vi "SLSC Write Properties.vi"(0 "session in":refnum<k21>, 1 "Stop Updating?":bool, 3 "Detect?":bool[](array[boolean]), 5 "SLSC Module Name":refnum<k21>, 9 "Values":dbl[](array[numeric]), 11 "error in":errorcluster, 12 "SLSC Dynamic Outputs":T1[](array[typedef])) -> (4 "session out":refnum<k21>, 6 "SLSC Module Name":refnum<k21>, 8 "LoopRate(ms)":u32=50, 15 "error out":errorcluster)   [LabVIEW 2015, in "SLSC CD Engine.lvlib"]
uses:
  SLSC CD Engine.lvlib
  SLSC Dynamic Channel.ctl
  SLSC Datatype.ctl
  <vilib>/SLSC/Commit Properties for Devices.vi
  <vilib>/SLSC/Set Generic Property (U64).vi
  <vilib>/SLSC/Set Generic Property (U32).vi
  <vilib>/SLSC/Set Generic Property (String).vi
  <vilib>/SLSC/Set Generic Property (I64).vi
  <vilib>/SLSC/Set Generic Property (I32).vi
  <vilib>/SLSC/Set Generic Property (DBL).vi
  <vilib>/SLSC/Set Generic Property (Bool).vi
  <vilib>/SLSC/SLSC.lvlib
  <vilib>/NI VeriStand/Custom Device Tools/Custom Device Utility Library/Custom Device Utility Library.lvlib
  SLSC CD Shared/SLSC CD Shared.lvlib
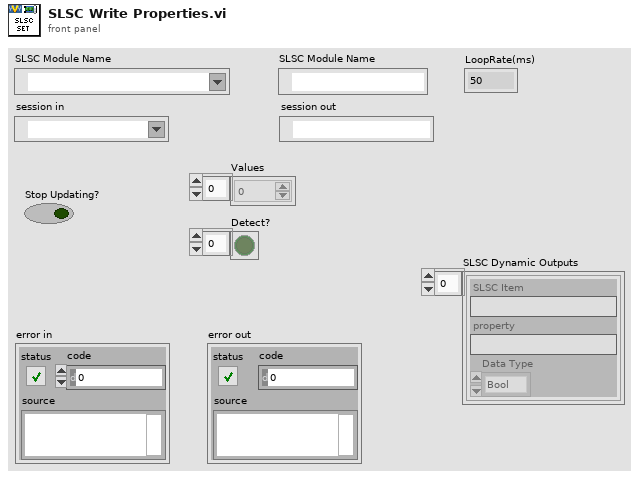
[diagram p1: front panel]
types:
  T1 = typedef "SLSC CD Shared.lvlib/SLSC Dynamic Channel.ctl" = cluster{"SLSC Item":string, "property":string, "Data Type":T2}
  T2 = typedef "SLSC CD Shared.lvlib/SLSC Datatype.ctl" = enum16{"Bool", "Double", "I32", "I64", "String", "U32", "U64"}
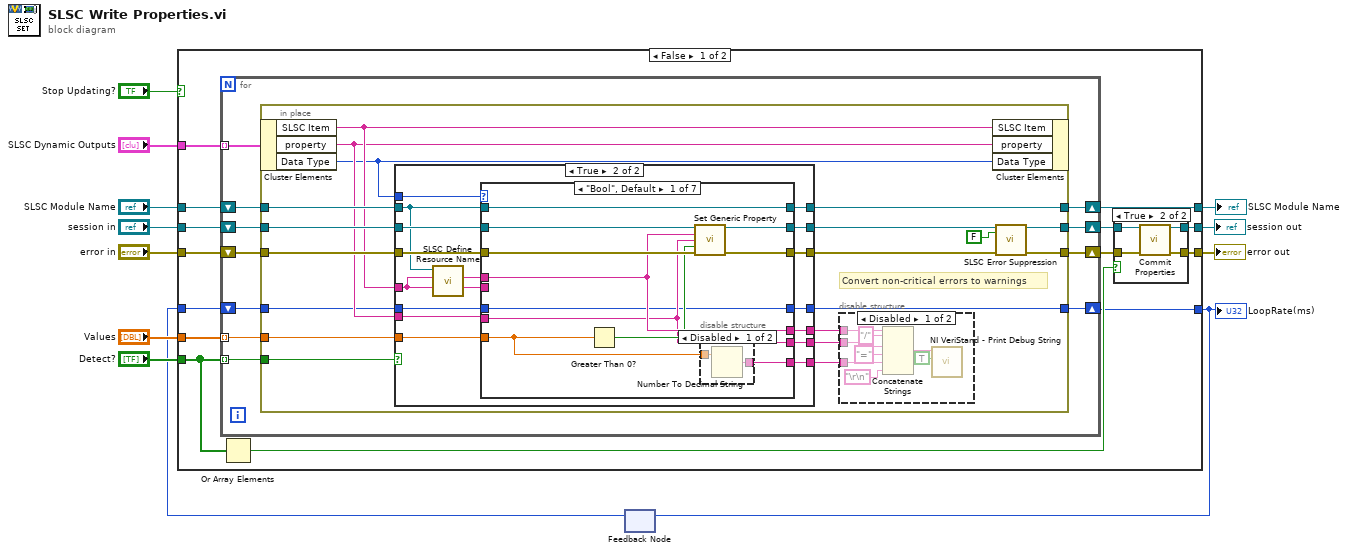
[diagram p0: block diagram]
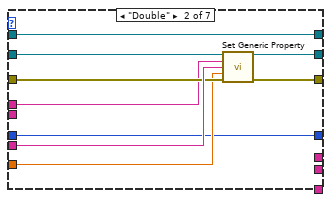
[diagram p6: hidden frame]
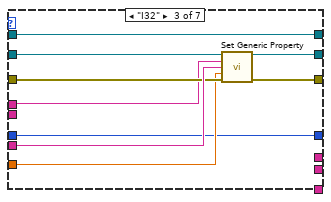
[diagram p7: hidden frame]
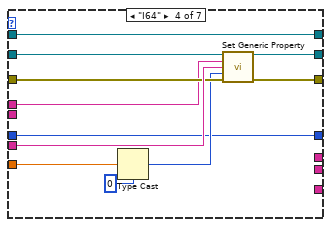
[diagram p8: hidden frame]
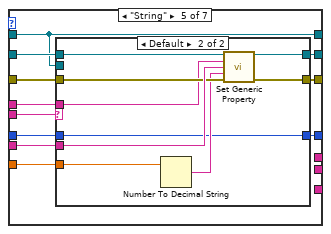
[diagram p9: hidden frame]
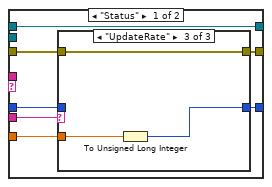
[diagram p10: hidden frame]
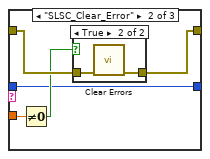
[diagram p12: hidden frame]
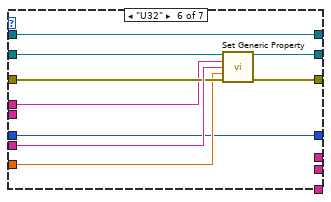
[diagram p14: hidden frame]
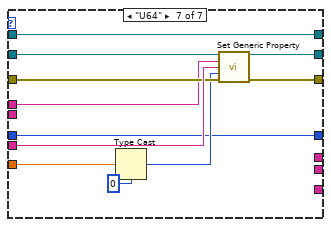
[diagram p15: hidden frame]
diagram:
  n1 = feedback #1() -> (w1:u32)  [unwired: 1 in]
  n2 = case shown="False" "Stop Updating?" {
    tunnel: "error in" -> [w26 w193]
    tunnel: "SLSC Dynamic Outputs" -> [w25 _]
    tunnel: "Values" -> [w24 _]
    tunnel: "session in" -> [w23 w194]
    tunnel: "SLSC Module Name" -> [w22 w195]
    tunnel: [w21 w195] -> w8
    tunnel: [w19 w193] -> w7
    tunnel: [w17 w194] -> w6
    tunnel: "Detect?" -> [w16 _]
    tunnel: [w13 w192] -> w2
    tunnel: w1 -> [w14 w192]
    frame False {
      n3 = for {
        tunnel: w24 -> [w43] mode=indexing
        tunnel: w25 -> [w36] mode=indexing
        shift-right: [w41] -> w18
        shift-left: w23 -> [w42]
        shift-right: [w40] -> w21
        shift-left: w22 -> [w37]
        tunnel: w16 -> [w35] mode=indexing
        shift-right: [w33] -> w13
        shift-left: w14 -> [w34]
        shift-right: [w38] -> w20
        shift-left: w26 -> [w39]
        n4 = in-place {
          in-place-border: w43 -> [w53]
          in-place-border: w42 -> [w61]
          in-place-border: [w60] -> w41
          in-place-border: [w59] -> w40
          in-place-border: w39 -> [w58]
          in-place-border: [w44] -> w38
          in-place-border: w37 -> [w57]
          in-place-border: w35 -> [w49]
          in-place-border: [w47] -> w33
          in-place-border: w34 -> [w46]
          # "Convert non-critical errors to warnings"
          n5 = in-place-cluster #2(w36) -> ("SLSC Item"=w56:string, "property"=w55:string, "Data Type"=w54:T2)
          n6 = case shown="True" w49 {
            tunnel: w61 -> [w72 w89]
            tunnel: [w72 w88] -> w60
            tunnel: [w73 w87] -> w59
            tunnel: w58 -> [w71 w86]
            tunnel: [w71 w85] -> w48
            tunnel: w57 -> [w73 w84]
            tunnel: w56 -> [_ w82]
            tunnel: w55 -> [_ w81]
            tunnel: w54 -> [_ w80]
            tunnel: w53 -> [_ w79]
            tunnel: [_ w78] -> w52
            tunnel: [_ w77] -> w51
            tunnel: [_ w76] -> w50
            tunnel: [w70 w75] -> w47
            tunnel: w46 -> [w70 w74]
            frame False {
            }
            frame True {
              n7 = call "SLSC Define Resource Name.vi"("SLSC Item"=w82, "SLSC Module Name"=w84) -> ("Resource"=w83:string)  [unwired: 9 in]
              n8 = case shown="\"Bool\", Default" w80 {
                tunnel: w79 -> [w95 w105 w114 w125 w137 w174 w184]
                tunnel: w89 -> [w100 w111 w120 w131 w142 w180 w191]
                tunnel: [w99 w110 w119 w130 w141 w179 w190] -> w88
                tunnel: w81 -> [w92 w109 w118 w129 w140 w178 w189]
                tunnel: w84 -> [w98 w108 w117 w128 w136 w177 w188]
                tunnel: [w98 w108 w117 w128 w136 w177 w188] -> w87
                tunnel: w86 -> [w97 w107 w116 w127 w139 w176 w187]
                tunnel: [w96 w106 w115 w126 w138 w175 w186] -> w85
                tunnel: w83 -> [w94 w104 w113 w122 w134 w173 w182]
                tunnel: w82 -> [_ _ _ _ w135 _ _]
                tunnel: [w94 _ _ _ _ _ _] -> w78
                tunnel: [w92 _ _ _ _ _ _] -> w77
                tunnel: [w91 _ _ _ _ _ _] -> w76
                tunnel: [w90 w103 w112 w121 w133 w172 w181] -> w75
                tunnel: w74 -> [w90 w103 w112 w121 w132 w172 w181]
                frame "Bool", Default {
                  n9 = Greater Than 0?(x=w95) -> (x > 0?=w93:bool)
                  n10 = call-poly <vilib>:"Set Generic Property.vi"("session in"=w100, "resources"=w94, "property"=w92, "property value"=w93, "error in (no error)"=w97) -> ("session out"=w99:refnum<k21>, "error out"=w96:errorcluster)  [unwired: 9 in]
                  n11 = disable-structure shown="Disabled" {
                    disable-tunnel: w95 -> [w102 _]
                    disable-tunnel: [w101 _] -> w91
                    frame Disabled {
                      n12 = Number To Decimal String(number=w102) -> (decimal integer string=w101:string)  [unwired: 1 in]
                    }
                    frame Enabled {
                    }
                  }
                }
                frame "Double" {
                  n13 = call-poly <vilib>:"Set Generic Property.vi"("session in"=w111, "resources"=w104, "property"=w109, "property value"=w105, "error in (no error)"=w107) -> ("session out"=w110:refnum<k21>, "error out"=w106:errorcluster)  [unwired: 9 in]
                }
                frame "I32" {
                  n14 = call-poly <vilib>:"Set Generic Property.vi"("session in"=w120, "resources"=w113, "property"=w118, "property value"=w114, "error in (no error)"=w116) -> ("session out"=w119:refnum<k21>, "error out"=w115:errorcluster)  [unwired: 9 in]
                }
                frame "I64" {
                  n15 = Type Cast(type=i64 0 ("property value"), x=w125) -> (*(type *) &x=w123:i64)
                  n16 = call-poly <vilib>:"Set Generic Property.vi"("session in"=w131, "resources"=w122, "property"=w129, "property value"=w123, "error in (no error)"=w127) -> ("session out"=w130:refnum<k21>, "error out"=w126:errorcluster)  [unwired: 9 in]
                }
                frame "String" {
                  n17 = case shown="Default" w135 {
                    tunnel: w142 -> [w149 w171]
                    tunnel: [w149 w170] -> w141
                    tunnel: w140 -> [w147 w169]
                    tunnel: w136 -> [_ _]
                    tunnel: w139 -> [w145 w168]
                    tunnel: [w146 w167] -> w138
                    tunnel: w137 -> [w148 w166]
                    tunnel: w134 -> [_ w164]
                    tunnel: [w144 w163] -> w133
                    tunnel: w132 -> [w143 w163]
                    frame "Status" {
                      n18 = case shown="\"UpdateRate\"" w147 {
                        tunnel: w148 -> [_ w154 w161]
                        tunnel: [w151 w155 w162] -> w146
                        tunnel: w145 -> [w151 w156 w162]
                        tunnel: [w150 w152 w160] -> w144
                        tunnel: w143 -> [w150 w152 _]
                        frame Default {
                        }
                        frame "SLSC_Clear_Error" {
                          n19 = Not Equal To 0?(x=w154) -> (x != 0?=w153:bool)
                          n20 = case shown="True" w153 {
                            tunnel: w156 -> [w157 w159]
                            tunnel: [w157 w158] -> w155
                            frame False {
                            }
                            frame True {
                              n21 = call <vilib>:"Clear Errors.vi"("error in (no error)"=w159) -> ("error out"=w158:errorcluster)  [unwired: 5 in, 1 out]
                            }
                          }
                        }
                        frame "UpdateRate" {
                          n22 = To Unsigned Long Integer(number=w161) -> (unsigned 32bit integer=w160:u32)
                        }
                      }
                    }
                    frame Default {
                      n23 = Number To Decimal String(number=w166) -> (decimal integer string=w165:string)  [unwired: 1 in]
                      n24 = call-poly <vilib>:"Set Generic Property.vi"("session in"=w171, "resources"=w164, "property"=w169, "property value"=w165, "error in (no error)"=w168) -> ("session out"=w170:refnum<k21>, "error out"=w167:errorcluster)  [unwired: 9 in]
                    }
                  }
                }
                frame "U32" {
                  n25 = call-poly <vilib>:"Set Generic Property.vi"("session in"=w180, "resources"=w173, "property"=w178, "property value"=w174, "error in (no error)"=w176) -> ("session out"=w179:refnum<k21>, "error out"=w175:errorcluster)  [unwired: 9 in]
                }
                frame "U64" {
                  n26 = Type Cast(type=u64 0 ("property value"), x=w184) -> (*(type *) &x=w183:u64)
                  n27 = call-poly <vilib>:"Set Generic Property.vi"("session in"=w191, "resources"=w182, "property"=w189, "property value"=w183, "error in (no error)"=w187) -> ("session out"=w190:refnum<k21>, "error out"=w186:errorcluster)  [unwired: 9 in]
                }
              }
            }
          }
          n28 = disable-structure shown="Disabled" {
            disable-tunnel: w51 -> [w64 _]
            disable-tunnel: w50 -> [w63 _]
            disable-tunnel: w52 -> [w62 _]
            frame Disabled {
              n29 = Concatenate Strings(w62, "/" ("string"), w64, "=" ("string"), w63, "\r\n") -> (w68:string)
              n30 = call <vilib>:"NI VeriStand - Print Debug String.vi"("Add to log file? (T)"=TRUE, "Message"=w68) -> ()  [unwired: 9 in, 1 out]
            }
            frame Enabled {
            }
          }
          n31 = in-place-cluster #2("SLSC Item"=w56, "property"=w55, "Data Type"=w54) -> ()  [unwired: 1 out]
          n32 = call "SLSC Error Suppression.vi"("error in (no error)"=w48, "Popup Error?"=FALSE) -> ("error out"=w44:errorcluster)  [unwired: 7 in, 1 out]
        }
      }
      n33 = Or Array Elements(Boolean array=w16) -> (logical OR=w15:bool)
      n34 = case shown="True" w15 {
        tunnel: w20 -> [w27 w32]
        tunnel: [w27 w31] -> w19
        tunnel: w18 -> [w28 w30]
        tunnel: [w28 w29] -> w17
        frame False {
        }
        frame True {
          n35 = call-poly <vilib>:"Commit Properties.vi"("session in"=w30, "error in (no error)"=w32) -> ("session out"=w29:refnum<k21>, "error out"=w31:errorcluster)  [unwired: 12 in]
        }
      }
    }
    frame True {
    }
  }
  "error out" <- w7
  "session out" <- w6
  "SLSC Module Name" <- w8
  "LoopRate(ms)" <- w2
  n36 = feedback-in #1(w2) -> ()
